vi "_090.vi"() -> ()   [LabVIEW 2020]
panel:
  out "x > y?":bool
  in  "Array":dbl[](array[numeric])
  # "Fundamentals"
  # "Which of the following statements will always be TRUE when this VI runs?"
  # "Answer :"
  # "Greater? Function"
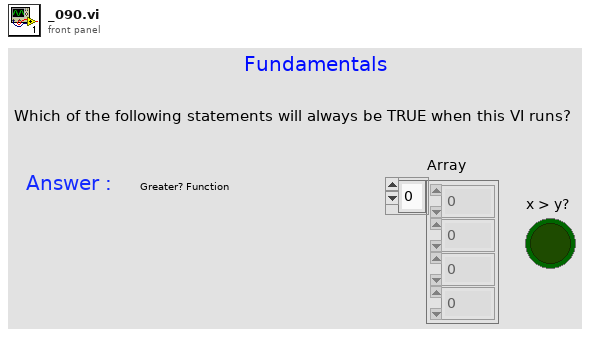
[diagram p1: front panel]
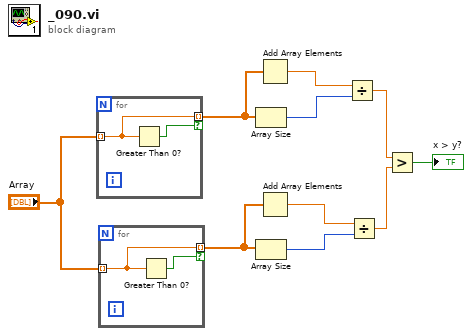
[diagram p0: block diagram]
diagram:
  n1 = for {
    tunnel: "Array" -> [w12] mode=indexing
    tunnel: [w12] -> w8 mode=indexing if=w11
    n2 = Greater Than 0?(x=w12) -> (x > 0?=w11:bool)
  }
  n3 = for {
    tunnel: "Array" -> [w14] mode=indexing
    tunnel: [w14] -> w9 mode=indexing if=w13
    n4 = Greater Than 0?(x=w14) -> (x > 0?=w13:bool)
  }
  n5 = Array Size(array=w8) -> (size(s)=w4:i32)
  n6 = Array Size(array=w9) -> (size(s)=w6:i32)
  n7 = Add Array Elements(numeric array=w8) -> (sum=w5:dbl)
  n8 = Add Array Elements(numeric array=w9) -> (sum=w7:dbl)
  n9 = Divide(x=w5, y=w4) -> (x/y=w3:dbl)
  n10 = Divide(x=w7, y=w6) -> (x/y=w2:dbl)
  n11 = Greater?(x=w3, y=w2) -> (0:→"x > y?":bool)
